vi "Station3_QR_Code_correct&localduplication_verification.vi"(9 "BARCODE STATION in":string, 10 "PART_NO":string, 11 "PRIVIOUS code":string[](array[string])) -> (2 "Correct part no True":bool, 3 "Correct part no & No duplication TRUE":bool)   [LabVIEW 2017]
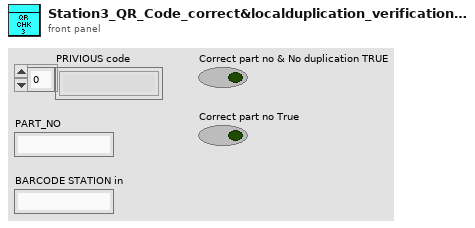
[diagram p1: front panel]
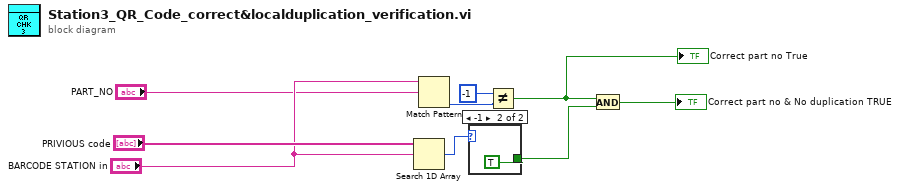
[diagram p0: block diagram]
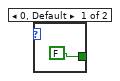
[diagram p2: hidden frame]
diagram:
  n1 = Search 1D Array(1D array="PRIVIOUS code", element="BARCODE STATION in") -> (index of element=w7:i32)  [unwired: 1 in]
  n2 = Match Pattern(string="BARCODE STATION in", regular expression="PART_NO") -> (offset past match=w3:i32)  [unwired: 1 in, 3 out]
  n3 = case shown="-1" w7 {
    tunnel: [FALSE TRUE] -> w8
    frame 0, Default {
    }
    frame -1 {
    }
  }
  n4 = Not Equal?(x=-1, y=w3) -> (x != y?=w1:bool)
  "Correct part no True" <- w1
  n5 = And(x=w1, y=w8) -> (x .and. y?=→"Correct part no & No duplication TRUE":bool)
